vi "isColored.vi"(0 "Camera in":refnum<class "Camera.lvclass">, 11 "error in (no error)":errorcluster) -> (4 "Camera out":refnum<class "Camera.lvclass">, 6 "colored":bool, 15 "error out":errorcluster)   [LabVIEW 2020, in "Camera.lvclass"]
doc: "Retreive the rec handle.\nThis handle allows direct access to all underlying functions of the pco.recorder."
uses:
  Camera.lvclass
  Camera.lvclass/Camera.ctl
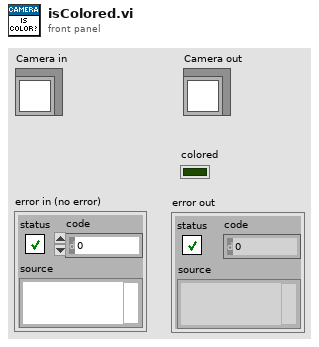
[diagram p1: front panel]
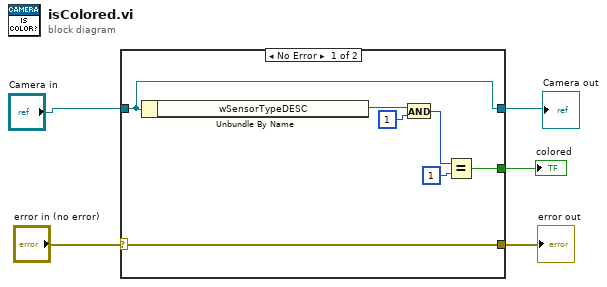
[diagram p0: block diagram]
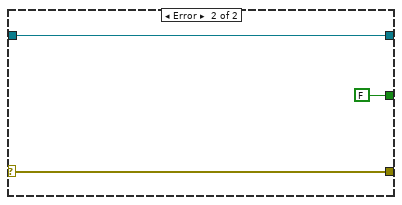
[diagram p2: hidden frame]
diagram:
  n1 = case shown="No Error" "error in (no error)" {
    selector: "error in (no error)" -> [w11 w15]
    tunnel: [w11 w15] -> w3
    tunnel: [w12 w14] -> w4
    tunnel: "Camera in" -> [w12 w14]
    tunnel: [w6 FALSE] -> w1
    frame No Error {
      n2 = Unbundle By Name(w12) -> ("wSensorTypeDESC"=w7:u16)
      n3 = And(x=w7, y=u16 1) -> (x .and. y?=w9:u16)
      n4 = Equal?(x=w9, y=u16 1) -> (x = y?=w6:bool)
    }
    frame Error {
    }
  }
  "error out" <- w3
  "Camera out" <- w4
  "colored" <- w1
